vi "2P_AdapUprite_Linlin.vi"() -> ()   [LabVIEW 2015] (continued)
                    n5185 = Equal?(x=w2192, y=-1.0) -> (x = y?=w2193:bool)
                    n5186 = case shown="False" w2193 {
                      tunnel: w2192 -> [w2218 _]
                      frame False {
                        n5187 = call "waveformparamsv2.vi"("command"="get") -> ("Params out"=w2201:T17)  [unwired: 4 in, 2 out]
                        n5188 = Unbundle By Name(w2201) -> ("AO parameters"=w2200:T18)
                        n5189 = Index Array(array=w2200, index=w2218) -> (element=w2217:T19)
                        n5190 = Unbundle By Name(w2217) -> ("AOtab"=w2198:dbl, "Repeats"=w2216:dbl, "Cycles"=w2215:dbl, "Start amplitude (V)"=w2214:dbl, "Baseline (V)"=w2213:dbl, "Step size (V)"=w2212:dbl, "DC (%)"=w2211:dbl, "Sampling frequency (Hz)"=w2210:dbl, "Period (ms)"=w2209:dbl, "Offset (V)"=w2208:dbl, "Amplitude (V)"=w2207:dbl, "Frequency"=w2206:dbl, "Tri Repeats"=w2205:dbl, "phase shift (ms)"=w2204:dbl, "Pulses"=w2203:dbl, "Tri phase"=w2199:dbl, "padding value"=w2195:dbl, "Matlab wave file"=w2196:path)
                        n5191 = To Unsigned Long Integer(number=w2198) -> (unsigned 32bit integer=w2197:u32)
                        n5192 = local write "Build analog waveform tabs"(w2197) -> ()
                        n5193 = local write "Matlab waveform path"(w2196) -> ()
                        n5194 = local write "phase shift (ms)"(w2204) -> ()
                        n5195 = local write "Repeats"(w2216) -> ()
                        n5196 = local write "Cycles"(w2215) -> ()
                        n5197 = local write "Amplitude (V)"(w2207) -> ()
                        n5198 = local write "Matlab padding value"(w2195) -> ()
                        n5199 = local write "Tri padding value"(w2195) -> ()
                        n5200 = local write "Start amplitude (V)"(w2214) -> ()
                        n5201 = local write "Tri Phase (s)"(w2199) -> ()
                        n5202 = local write "Period (ms)"(w2209) -> ()
                        n5203 = local write "Tri Repeats"(w2205) -> ()
                        n5204 = local write "Offset (V)"(w2208) -> ()
                        n5205 = local write "Frequency"(w2206) -> ()
                        n5206 = local write "Pulses"(w2203) -> ()
                        n5207 = local write "padding value"(w2195) -> ()
                        n5208 = local write "Sampling rate \ncurrent wf"(w2210) -> ()
                        n5209 = local write "Baseline (V)"(w2213) -> ()
                        n5210 = local write "Step size (V)"(w2212) -> ()
                        n5211 = local write "DC (%)"(w2211) -> ()
                      }
                      frame True {
                      }
                    }
                  }
                  frame #5 {
                    n5212 = local read "DO channels"() -> (w2221:u16)
                    n5213 = call "2pparameters.vi"("command"="get") -> ("params out"=w2223:T12)  [unwired: 1 in]
                    n5214 = Unbundle By Name(w2223) -> ("aDO"=w2222:u32[])
                    n5215 = Search 1D Array(1D array=w2222, element=w2221) -> (index of element=w2220:i32)  [unwired: 1 in]
                    n5216 = Equal?(x=w2220, y=-1.0) -> (x = y?=w2219:bool)
                    n5217 = case shown="False" w2219 {
                      tunnel: w2220 -> [w2238 _]
                      frame False {
                        n5218 = call "waveformparamsv2.vi"("command"="get") -> ("Params out"=w2232:T17)  [unwired: 4 in, 2 out]
                        n5219 = Unbundle By Name(w2232) -> ("DO parameters"=w2230:T20)
                        n5220 = Index Array(array=w2230, index=w2238) -> (element=w2237:T21)
                        n5221 = Unbundle By Name(w2237) -> ("Digital DC (%)"=w2236:dbl, "Digital phase"=w2235:dbl, "Digital Freq (Hz)"=w2234:dbl, "Sampling frequency (Hz)"=w2233:dbl, "Digital time offset (s)"=w2229:dbl, "padding value"=w2228:dbl, "matlab wave file"=w2227:path, "DOtab"=w2226:dbl)
                        n5222 = local write "Build digital waveform tabs"(w2226) -> ()
                        n5223 = local write "Digital DC (%)"(w2236) -> ()
                        n5224 = local write "Matlab waveform path DO"(w2227) -> ()
                        n5225 = local write "Sampling rate \ncurrent wf"(w2233) -> ()
                        n5226 = local write "Digital time offset (s)"(w2229) -> ()
                        n5227 = local write "Matlab padding value DO"(w2228) -> ()
                        n5228 = local write "Digital padding value"(w2228) -> ()
                        n5229 = local write "Digital Freq (Hz)"(w2234) -> ()
                        n5230 = local write "Digital phase (s)"(w2235) -> ()
                      }
                      frame True {
                      }
                    }
                  }
                  frame #6 {
                    n5231 = local read "finite samples"() -> (w2240:bool)
                    n5232 = local read "continuous"() -> (w2241:bool)
                    n5233 = local read "wavdet"() -> (w2242:bool)
                    n5234 = call "2pparameters.vi"("command"="get") -> ("params out"=w2245:T12)  [unwired: 1 in]
                    n5235 = Bundle By Name(cluster=w2245, "finite"=w2240, "cont"=w2241, "wavdet"=w2242) -> (w2243:T12)
                    n5236 = property on="Update settings" class="Bool (strict)"("Val(Sgnl)"=FALSE ("Value (Signaling)")) -> ()  [unwired: 2 in, 2 out]
                    n5237 = call "2pparameters.vi"("Params in"=w2243, "command"="set") -> ()  [unwired: 1 out]
                  }
                }
              }
            }
          }
          event "Digital phase (s)", "Digital DC (%)", "Digital Freq (Hz)", "Digital padding value", "Digital time offset (s)": Value Change {
            n5238 = event-data() -> ()  [unwired: 1 in, 6 out]
            n5239 = local write "not loadedDO"(TRUE ("not loadedDO")) -> ()
          }
          event "Matlab padding value DO", "Matlab waveform path DO": Value Change {
            n5240 = event-data() -> ()  [unwired: 1 in, 6 out]
            n5241 = local write "not loadedDOml"(TRUE ("not loadedDO")) -> ()
          }
          event "phase shift (ms)", "Pulses", "Baseline (V)", "Step size (V)", "Start amplitude (V)", "Period (ms)", "DC (%)", "Cycles", "Repeats", "padding value": Value Change {
            n5242 = event-data() -> ()  [unwired: 1 in, 6 out]
            n5243 = local write "not loaded"(TRUE ("not loaded")) -> ()
          }
          event "Tri Repeats", "Amplitude (V)", "Offset (V)", "Frequency", "Tri Phase (s)", "Tri padding value": Value Change {
            n5244 = event-data() -> ()  [unwired: 1 in, 6 out]
            n5245 = local write "not loadedtri"(TRUE ("not loadedtri")) -> ()
          }
          event "Matlab waveform path", "Matlab padding value": Value Change {
            n5246 = event-data() -> ()  [unwired: 1 in, 6 out]
            n5247 = local write "not loadedml"(TRUE ("not loadedml")) -> ()
          }
          event "Exit": Value Change {
            n5248 = event-data() -> ("NewVal"=w2252:bool)  [unwired: 1 in]
          }
        }
        n5249 = Wait (ms)(milliseconds to wait=u32 50) -> ()  [unwired: 1 out]
      }
    }
    frame #3 {
      w6897 = FALSE ("Value (Signaling)")
      n5250 = property on="Start" class="Bool (strict)"("Val(Sgnl)"=w6897) -> ()  [unwired: 2 in, 2 out]
      n5251 = property on="Exit" class="Bool (strict)"("Val(Sgnl)"=w6897) -> ()  [unwired: 2 in, 2 out]
      n5252 = property on="Stop" class="Bool (strict)"("Val(Sgnl)"=w6897) -> ()  [unwired: 2 in, 2 out]
      n5253 = flat-sequence {
        frame #0 {
          n5254 = disable-structure shown="Disabled" {
            frame Disabled {
              w6898 = u16 1 items=["OD 0"=1, "OD 0.5"=2, "OD 1"=3, "OD 2"=4, "OD 3"=5, "OD 4"=6] ("New ODfilt")
              n5255 = local read "ODfilt"() -> (w6899:u16)
              n5256 = call "filterwheelcontrol_nothorlabslib.vi"("Current OD filt"=w6899, "New ODfilt"=w6898) -> ()  [unwired: 1 in]
            }
            frame Enabled {
            }
          }
        }
        frame #1 {
          n5257 = Wait (ms)(milliseconds to wait=u32 1000) -> ()  [unwired: 1 out]
        }
      }
    }
  }
